vi "Asynchronous - Update RTs Status.vi"(5 "Raw Values (RTs Status)":T3, 7 "Map (RTs Status)":T1[](array[typedef]), 8 "Error (in)":errorcluster, 9 "Updated FIFO Index []":i32[](array[numeric]), 10 "U16 []":u16[](array[numeric])) -> (0 "Error (out)":errorcluster)   [LabVIEW 2017, in "Ballard MIL-1553 Engine.lvlib"]
uses:
  Ballard MIL-1553 Engine.lvlib
  Controls/RT Async_Raw Values.ctl
  Controls/RT Async_Raw Values to Messages Index_Association.ctl
  Controls/RT Async_Map RTs Status.ctl
  Controls/RT Async_Map_Type.ctl
  <instrlib>/BTI1553Lib/BTI1553LV.lvlib
  <vilib>/NI VeriStand/Custom Device Tools/Custom Device Utility Library/Custom Device Utility Library.lvlib
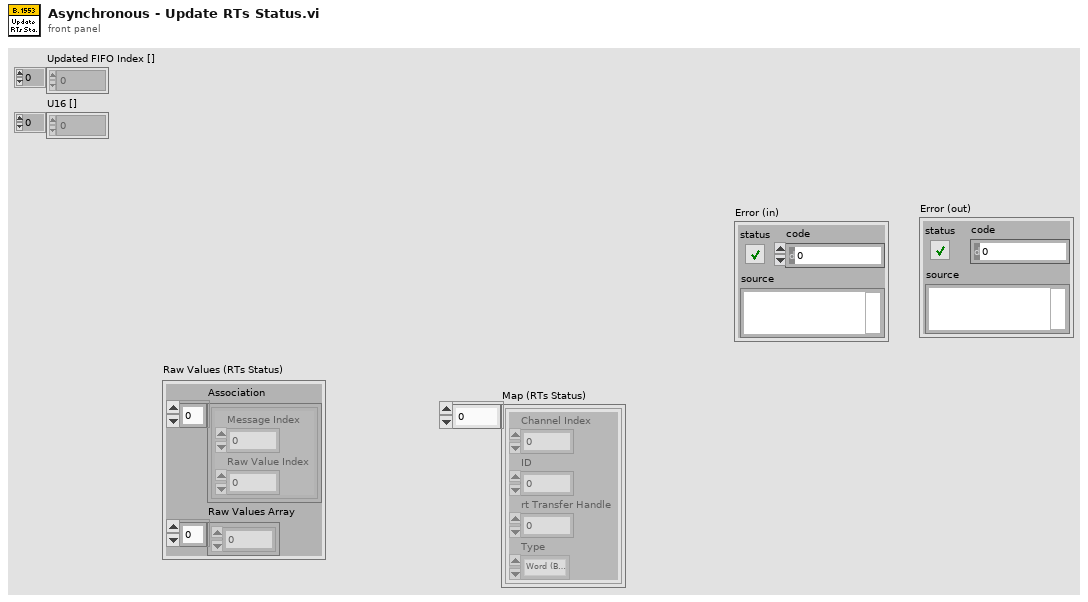
[diagram p1: front panel]
types:
  T1 = typedef "Ballard MIL-1553 Engine.lvlib/RT Async_Map RTs Status.ctl" = cluster{"Channel Index":i32, "ID":i32, "rt Transfer Handle":u64, "Type":T2}
  T2 = typedef "Ballard MIL-1553 Engine.lvlib/RT Async_Map_Type.ctl" = enum16{"Word (BC to RT)", "Word (MC (Rx))", "Acyclic Message Trigger", "Word (RT to ..)", "Word (RT to RT)", "Word (MC (Tx))", "RT Status", "BC Commands", "RT Commands"}
  T3 = typedef "Ballard MIL-1553 Engine.lvlib/RT Async_Raw Values.ctl" = cluster{"Association":T4[], "Raw Values Array":u16[]}
  T4 = typedef "Ballard MIL-1553 Engine.lvlib/RT Async_Raw Values to Messages Index_Association.ctl" = cluster{"Message Index":i32, "Raw Value Index":i32}
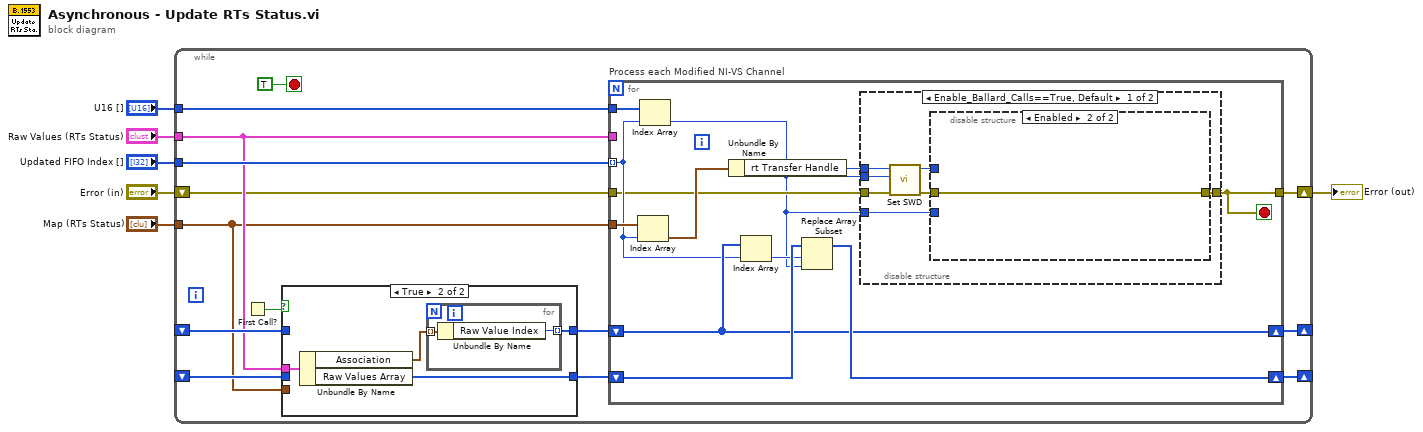
[diagram p0: block diagram]
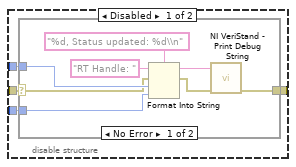
[diagram p3: hidden frame]
diagram:
  n1 = while {
    tunnel: "Raw Values (RTs Status)" -> [w11]
    tunnel: "Updated FIFO Index []" -> [w20]
    tunnel: "U16 []" -> [w19]
    tunnel: "Map (RTs Status)" -> [w10]
    shift-right: [w8] -> w3
    shift-left: "Error (in)" -> [w7]
    shift-right: [w9] -> _
    shift-left: _ -> [w16]
    shift-right: [w14] -> _
    shift-left: _ -> [w13]
    stop <- TRUE stop-if-true
    n2 = First Call?() -> (First Call?: T/F=w12:bool)
    n3 = case shown="True" w12 {
      tunnel: w11 -> [_ w26]
      tunnel: [w22 w25] -> w17
      tunnel: w16 -> [w22 _]
      tunnel: [w21 w23] -> w15
      tunnel: w13 -> [w21 _]
      tunnel: w10 -> [_ _]
      frame False {
      }
      frame True {
        n4 = Unbundle By Name(w26) -> ("Association"=w24:T4[], "Raw Values Array"=w25:u16[])
        n5 = for {
          tunnel: w24 -> [w28] mode=indexing
          tunnel: [w27] -> w23 mode=indexing
          n6 = Unbundle By Name(w28) -> ("Raw Value Index"=w27:i32)
        }
      }
    }
    n7 = for "Process each Modified NI-VS Channel" {
      tunnel: w11 -> [_]
      tunnel: w20 -> [w35] mode=indexing
      tunnel: w19 -> [w39]
      tunnel: w7 -> [w31]
      tunnel: [w30] -> w8
      tunnel: w10 -> [w40]
      shift-right: [w37] -> w9
      shift-left: w17 -> [w38]
      shift-right: [w36] -> w14
      shift-left: w15 -> [w36]
      stop <- w30 stop-if-true
      n8 = Index Array(array=w40, index=w35) -> (element=w33:T1)
      n9 = Index Array(array=w39, index=w35) -> (element=w29:u16)
      n10 = Unbundle By Name(w33) -> ("rt Transfer Handle"=w32:u64)
      n11 = Index Array(array=w36, index=w35) -> (element=w34:i32)
      n12 = Replace Array Subset(array=w38, new element=w29, index=w34) -> (w37:u16[])
      n13 = disable-structure shown="Enable_Ballard_Calls==True, Default" {
        disable-tunnel: w32 -> [w47 _]
        disable-tunnel: w31 -> [w46 w62]
        disable-tunnel: [w42 w62] -> w30
        disable-tunnel: w29 -> [w45 _]
        disable-tunnel: w29 -> [w41 _]
        frame condition #0 (active) {
          n14 = call <instrlib>:"Set SWD.vi"("error in (no error)"=w46, "status word"=w45, "remote terminal handle in"=w47) -> ("error out"=w44:errorcluster, "remote terminal handle out"=w43:u64)  [unwired: 7 in]
          n15 = disable-structure shown="Enabled" {
            disable-tunnel: w44 -> [w51 w61]
            disable-tunnel: w43 -> [w50 _]
            disable-tunnel: [w49 w61] -> w42
            disable-tunnel: w41 -> [w48 _]
            frame Disabled {
              n16 = case shown="No Error" w51 {
                selector: w51 -> [w53 w60]
                tunnel: [w58 w60] -> w49
                tunnel: w50 -> [w55 _]
                tunnel: w48 -> [w52 _]
                frame No Error {
                  n17 = Format Into String(format string="%d, Status updated: %d\\n", initial string="RT Handle: ", error in=w53, w55, w52) -> (resulting string=w59:string, error out=w54:errorcluster)
                  n18 = call <vilib>:"NI VeriStand - Print Debug String.vi"("error in (no error)"=w54, "Message"=w59) -> ("error out"=w58:errorcluster)  [unwired: 9 in]
                }
                frame Error {
                }
              }
            }
            frame Enabled {
            }
          }
        }
        frame condition #1 {
        }
      }
    }
  }
  "Error (out)" <- w3
